vi "Initiate SMU Trigger Model.vi"(8 "error in (no error)":errorcluster, 10 "Source Measure Unit Channel (0: Channel A)":i32(ring) items=["Channel A", "Channel B"], 11 "VISA resource name":refnum<visa-resource-name>) -> (0 "error out":errorcluster, 3 "VISA resource name out":refnum<visa-resource-name>)   [LabVIEW 2015, in "Keithley 2600 Series.lvlib"]
doc: "Initiates a preconfigured sweep and clears the event detectors for source measure unit channel.\n\n<b>Note:</b>\nYou must turn on the source output by <b>Enable Source Output </b>VI before you call this VI."
uses:
  Keithley 2600 Series.lvlib
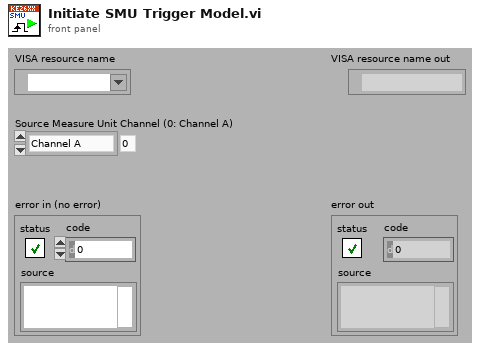
[diagram p1: front panel]
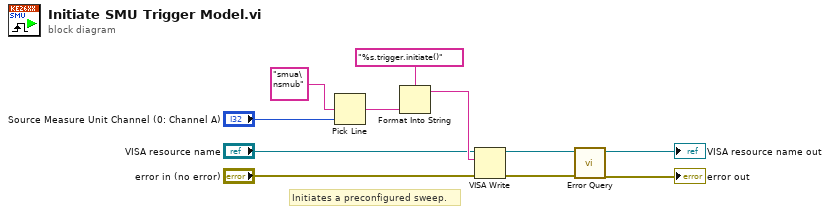
[diagram p0: block diagram]
diagram:
  # "Initiates a preconfigured sweep."
  n1 = Pick Line(multi-line string="smua\nsmub", line index="Source Measure Unit Channel (0: Channel A)") -> (output string=w1:string)  [unwired: 1 in]
  n2 = Format Into String(format string="%s.trigger.initiate()", w1) -> (resulting string=w10:string)  [unwired: 2 in, 1 out]
  n3 = VISA Write(VISA resource name="VISA resource name", write buffer=w10, error in (no error)="error in (no error)") -> (VISA resource name out=w7:refnum<visa-resource-name>, error out=w6:errorcluster)  [unwired: 1 out]
  n4 = call "Error Query.vi"("error in (no error)"=w6, "VISA resource name"=w7) -> ("error out"=→"error out":errorcluster, "VISA resource name out"=→"VISA resource name out":refnum<visa-resource-name>)  [unwired: 6 in, 2 out]
